vi "Create All Blocks.vi"(8 "error in (no error)":errorcluster, 10 "Grid":refnum<data-value>, 11 "Board in":refnum<class "Board.lvclass">) -> (0 "error out":errorcluster, 2 "New Blocks":refnum<data-value>[](array[refnum]), 3 "Board out":refnum<class "Board.lvclass">)   [LabVIEW 2017, in "Board.lvclass"]
uses:
  Board.lvclass
  <vilib>/LIEF/Forms/Shape/Shape.lvclass
  Board.lvclass/Board.ctl
  Block/Block.lvclass
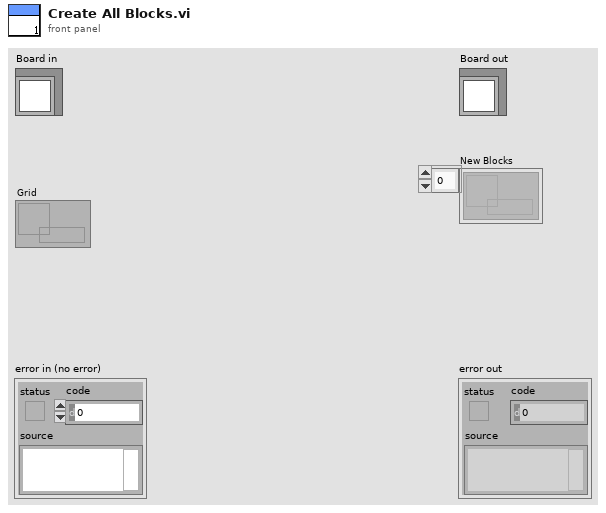
[diagram p1: front panel]
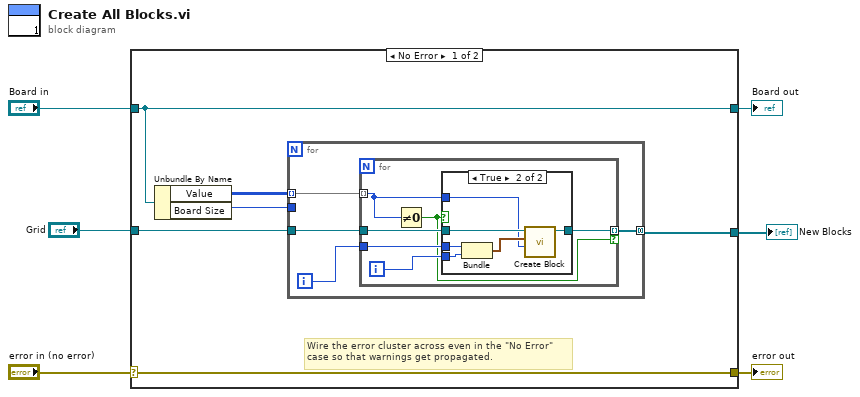
[diagram p0: block diagram]
diagram:
  n1 = case shown="No Error" "error in (no error)" {
    selector: "error in (no error)" -> [w12 w30]
    tunnel: [w12 w30] -> w5
    tunnel: [w11 w29] -> w3
    tunnel: "Board in" -> [w11 w29]
    tunnel: "Grid" -> [w10 _]
    tunnel: [w7 _] -> w1
    frame No Error {
      # "Wire the error cluster across even in the \"No Error\"\ncase so that warnings get propagated."
      n2 = Unbundle By Name(w11) -> ("Value"=w9:u32[][], "Board Size"=w8:u16)
      n3 = for {
        tunnel: w10 -> [w16]
        tunnel: w9 -> [w15] mode=indexing
        tunnel: w8 -> [_]
        tunnel: [w13] -> w7 mode=concatenating
        i -> [w14]
        n4 = for {
          tunnel: w16 -> [w22]
          tunnel: w15 -> [w19] mode=indexing
          tunnel: w14 -> [w21]
          tunnel: [w18] -> w13 mode=indexing if=w17
          i -> [w20]
          n5 = Not Equal To 0?(x=w19) -> (x != 0?=w17:bool)
          n6 = case shown="True" w17 {
            tunnel: w22 -> [_ w28]
            tunnel: w21 -> [_ w27]
            tunnel: w20 -> [_ w26]
            tunnel: w19 -> [_ w23]
            tunnel: [_ w24] -> w18
            frame False {
            }
            frame True {
              n7 = Bundle(w27, w26) -> (w25:cluster{i32, i32})  [unwired: 1 in]
              n8 = call "Create Block.vi"("Value"=w23, "Available Indexes"=w25, "Grid"=w28) -> ("New Block"=w24:refnum<data-value>)  [unwired: 7 in, 1 out]
            }
          }
        }
      }
    }
    frame Error {
    }
  }
  "error out" <- w5
  "Board out" <- w3
  "New Blocks" <- w1
